vi "Close.vi"(8 "Error In":errorcluster, 11 "PS4 Controller Ref":T1) -> (0 "Error Out":errorcluster)   [LabVIEW 2020, in "LMH-PS4.lvlib"]
doc: "Close the connection to the PS4 controller."
uses:
  LMH-PS4.lvlib
  Private/Type Defs/PS4 Controller Ref.ctl
  <vilib>/Utility/inputDevices.llb/closeJoystick.vi
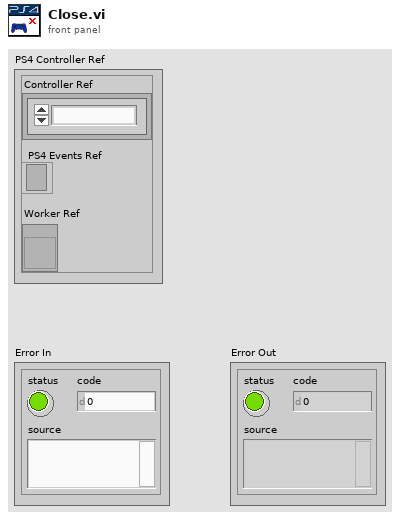
[diagram p1: front panel]
types:
  T1 = typedef "LMH-PS4.lvlib/PS4 Controller Ref.ctl" = cluster{"Controller Ref":refnum<k1>, "PS4 Events Ref":refnum<event-registration>, "Worker Ref":refnum<vi>}
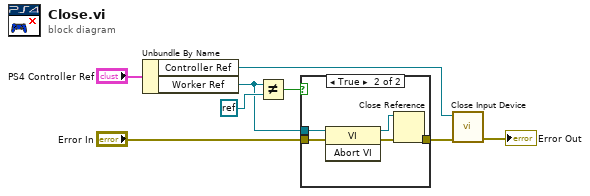
[diagram p0: block diagram]
diagram:
  n1 = Unbundle By Name("PS4 Controller Ref") -> ("Controller Ref"=w5:refnum<k1>, "Worker Ref"=w2:refnum<vi>)
  n2 = Not Equal?(x=w2, y=refnum<k0> refnum) -> (x != y?=w3:bool)
  n3 = case shown="True" w3 {
    tunnel: [w9 w12] -> w8
    tunnel: "Error In" -> [w9 w11]
    tunnel: w2 -> [_ w10]
    frame False {
      # "Worker Not \nEnabled"
    }
    frame True {
      n4 = invoke class="VI" method="Abort VI"(reference=w10, error in=w11) -> (reference out=w13:refnum<vi>, error out=w14:errorcluster)  [unwired: 1 in, 1 out]
      n5 = Close Reference(reference=w13, error in (no error)=w14) -> (error out=w12:errorcluster)
    }
  }
  n6 = call-poly <vilib>:"Close Input Device.vi"("error in (no error)"=w8, "device ID"=w5) -> ("error out"=→"Error Out":errorcluster)  [unwired: 8 in]
